vi "VI Get All Input.vi"(8 "error in (no error)":errorcluster, 11 "CallVIStep in":refnum<class "CallVIStep.lvclass">) -> (0 "error out":errorcluster, 2 "Input Control":T1[](array[typedef]), 3 "CallVIStep out":refnum<class "CallVIStep.lvclass">)   [LabVIEW 2015, in "CallVIStep.lvclass"]
uses:
  CallVIStep.lvclass
  VI Input Control Typedef.ctl
  VI Input Type Typedef.ctl
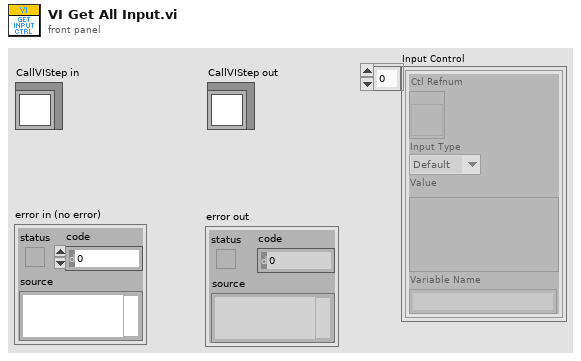
[diagram p1: front panel]
types:
  T1 = typedef "CallVIStep.lvclass/VI Input Control Typedef.ctl" = cluster{"Ctl Refnum":refnum<vi>, "Input Type":T2, "Value":variant, "Variable Name":string}
  T2 = typedef "CallVIStep.lvclass/VI Input Type Typedef.ctl" = enum16{"Default", "Value", "Variable"}
  T3 = typedef "CallVIStep.lvclass/VI Input Typedef.ctl" = cluster{"Label":string, "Input Type":T2, "Type String":i16[], "Data String":string, "Variable Name":string}
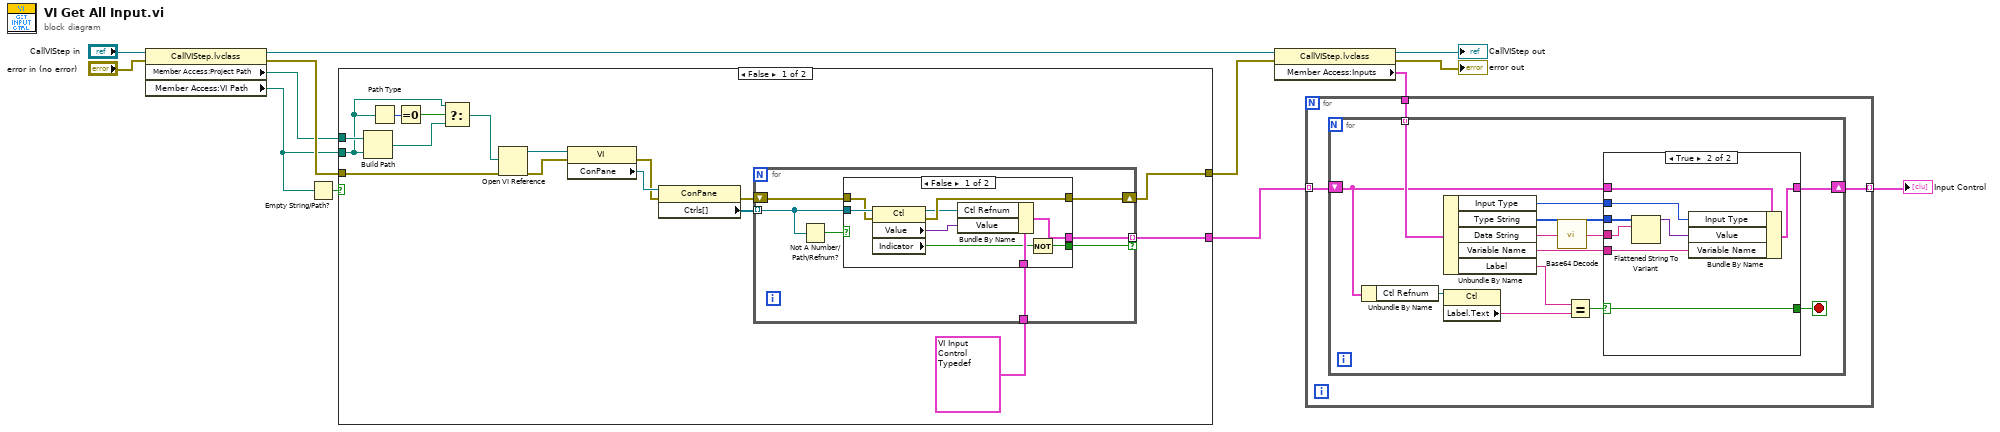
[diagram p0: block diagram]
diagram:
  n1 = property class="CallVIStep.lvclass"(reference="CallVIStep in", error in="error in (no error)") -> (reference out=w9:refnum<class "CallVIStep.lvclass">, error out=w12:errorcluster, "Member Access:Project Path"=w2:path, "Member Access:VI Path"=w1:path)
  n2 = Empty String/Path?(string/path=w1) -> (empty?=w10:bool)
  n3 = case shown="False" w10 {
    tunnel: w12 -> [w29 w47]
    tunnel: [w21 _] -> w5
    tunnel: w1 -> [w16 _]
    tunnel: [w20 w47] -> w7
    tunnel: w2 -> [w19 _]
    frame False {
      n4 = Build Path(base path=w19, name or relative path=w16) -> (appended path=w15:path)
      n5 = Path Type(1:w16) -> (0:w18:i16)
      n6 = Equal To 0?(x=w18) -> (x = 0?=w17:bool)
      n7 = Select(t=w16, s=w17, f=w15) -> (s? t:f=w14:path)
      n8 = Open VI Reference(vi path=w14, error in (no error)=w29) -> (vi reference=w26:refnum<vi>, error out=w25:errorcluster)  [unwired: 4 in]
      n9 = property class="VI"(reference=w26, error in=w25) -> (error out=w24:errorcluster, "ConPane"=w28:refnum<vi>)  [unwired: 1 out]
      n10 = property class="ConPane"(reference=w28, error in=w24) -> (error out=w23:errorcluster, "Ctrls[]"=w27:refnum<vi>[])  [unwired: 1 out]
      n11 = for {
        tunnel: w27 -> [w31] mode=indexing
        tunnel: [w35] -> w21 mode=indexing if=w30
        shift-right: [w32] -> w20
        shift-left: w23 -> [w34]
        tunnel: T1 {"Ctl Refnum"=refnum, "Input Type"=enum."Default", "Value"=variant, "Variable Name"=""} -> [w33]
        n12 = Not A Number/Path/Refnum?(number/path/refnum=w31) -> (NaN/Path/Refnum?=w36:bool)
        n13 = case shown="False" w36 {
          tunnel: w31 -> [w45 _]
          tunnel: [w44 _] -> w35
          tunnel: [w37 _] -> w30
          tunnel: w34 -> [w43 w46]
          tunnel: w33 -> [w42 _]
          tunnel: [w41 w46] -> w32
          frame False {
            n14 = property class="Ctl"(reference=w45, error in=w43) -> (reference out=w40:refnum<vi>, error out=w41:errorcluster, "Value"=w39:variant, "Indicator"=w38:bool)
            n15 = Bundle By Name(cluster=w42, "Ctl Refnum"=w40, "Value"=w39) -> (w44:T1)
            n16 = Not(x=w38) -> (.not. x?=w37:bool)
          }
          frame True {
          }
        }
      }
    }
    frame True {
    }
  }
  n17 = property class="CallVIStep.lvclass"(reference=w9, error in=w7) -> (reference out=→"CallVIStep out":refnum<class "CallVIStep.lvclass">, error out=→"error out":errorcluster, "Member Access:Inputs"=w4:T3[])
  n18 = for {
    tunnel: w5 -> [w49] mode=indexing
    tunnel: w4 -> [w50]
    tunnel: [w48] -> w3 mode=indexing
    n19 = for {
      tunnel: w50 -> [w62] mode=indexing
      shift-right: [w59] -> w48
      shift-left: w49 -> [w60]
      stop <- w58 stop-if-true
      n20 = Unbundle By Name(w60) -> ("Ctl Refnum"=w63:refnum<vi>)
      n21 = Unbundle By Name(w62) -> ("Input Type"=w57:T2, "Type String"=w56:i16[], "Data String"=w55:string, "Variable Name"=w51:string, "Label"=w52:string)
      n22 = property class="Ctl"(reference=w63) -> ("Label.Text"=w61:string)  [unwired: 1 in, 2 out]
      n23 = call "Base64 Decode.vi"("base64 string"=w55) -> ("normal string"=w54:string)
      n24 = Equal?(x=w52, y=w61) -> (x = y?=w53:bool)
      n25 = case shown="True" w53 {
        selector: w53 -> [w65 w71]
        tunnel: w60 -> [w64 w73]
        tunnel: w54 -> [_ w68]
        tunnel: [w64 w72] -> w59
        tunnel: [w65 w71] -> w58
        tunnel: w57 -> [_ w70]
        tunnel: w56 -> [_ w69]
        tunnel: w51 -> [_ w66]
        frame False {
        }
        frame True {
          n26 = Flattened String To Variant(6:w68, 7:w69) -> (3:w67:variant)  [unwired: 1 in, 1 out]
          n27 = Bundle By Name(cluster=w73, "Input Type"=w70, "Value"=w67, "Variable Name"=w66) -> (w72:T1)
        }
      }
    }
  }
  "Input Control" <- w3
